vi "load.vi"(8 "error in (no error)":errorcluster, 11 "Notebook in":refnum<class "Notebook.lvclass">) -> (0 "error out":errorcluster, 3 "Notebook out":refnum<class "Notebook.lvclass">)   [LabVIEW 2010, in "Notebook.lvclass"]
uses:
  Notebook.lvclass
  Notebook.lvclass/Notebook.ctl
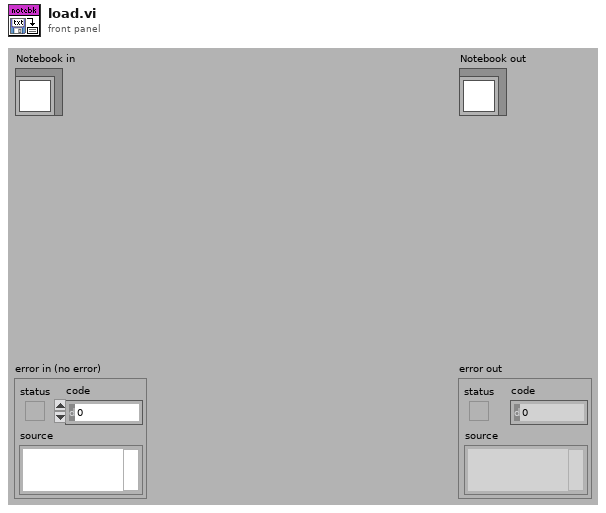
[diagram p1: front panel]
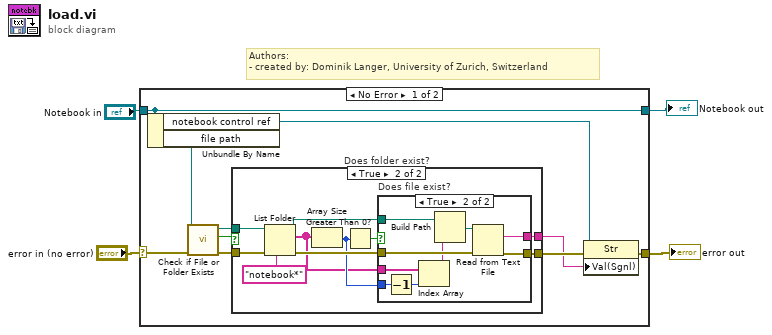
[diagram p0: block diagram]
diagram:
  # "Authors: \n- created by: Dominik Langer, University of Zurich, Switzerland"
  n1 = case shown="No Error" "error in (no error)" {
    selector: "error in (no error)" -> [w9 w37]
    tunnel: [w13 w37] -> w3
    tunnel: [w14 w36] -> w1
    tunnel: "Notebook in" -> [w14 w36]
    frame No Error {
      n2 = Unbundle By Name(w14) -> ("notebook control ref"=w11:refnum<vi>, "file path"=w7:path)
      n3 = call <vilib>:"Check if File or Folder Exists.vi"("error in (no error)"=w9, "path"=w7) -> ("error out"=w8:errorcluster, "file or folder exists?"=w5:bool, "dup path"=w6:path)  [unwired: 7 in]
      n4 = case "Does folder exist?" shown="True" w5 {
        tunnel: [w15 w25] -> w12
        tunnel: [_ w24] -> w10
        tunnel: w8 -> [w15 w18]
        tunnel: w6 -> [_ w17]
        frame False {
        }
        frame True {
          n5 = List Folder(path=w17, pattern="notebook*", error in=w18) -> (path out=w16:path, filenames=w19:string[], error out=w21:errorcluster)  [unwired: 1 in, 1 out]
          n6 = Array Size(array=w19) -> (size(s)=w20:i32)
          n7 = Greater Than 0?(x=w20) -> (x > 0?=w22:bool)
          n8 = case "Does file exist?" shown="True" w22 {
            tunnel: [w26 w35] -> w25
            tunnel: [_ w34] -> w24
            tunnel: w21 -> [w26 w33]
            tunnel: w16 -> [_ w29]
            tunnel: w20 -> [_ w32]
            tunnel: w19 -> [_ w30]
            frame False {
            }
            frame True {
              n9 = Decrement(x=w32) -> (x-1=w31:i32)
              n10 = Index Array(array=w30, index=w31) -> (element=w28:string)
              n11 = Build Path(base path=w29, name or relative path=w28) -> (appended path=w27:path)
              n12 = Read from Text File(file (use dialog)=w27, error in=w33) -> (text=w34:string, error out=w35:errorcluster)  [unwired: 4 out]
            }
          }
        }
      }
      n13 = property class="Str"(reference=w11, error in=w12, "Val(Sgnl)"=w10) -> (error out=w13:errorcluster)  [unwired: 1 out]
    }
    frame Error {
    }
  }
  "error out" <- w3
  "Notebook out" <- w1
